vi "Start WiFi with DHCP.vi"(7 "Retry wait time [ms]":u32=100, 8 "Error In":errorcluster, 11 "LINX Resource":T2) -> (0 "error out":errorcluster, 2 "TCP Configuration Out":T1, 3 "LINX Resource Out":T2={"IO"=enum."Remote", "Interface"=enum."Serial", "LINX Device Config"={"Interface"=enum."Serial", "COM Port"="COM13", "TCP Configuration"={"IP Address"="", "Port"=0}, "Device Family"=1, "Device ID"=1, "Device Name"="myRIO-1900", "TCP Ref"=refnum, "Channels"={"DI"=[0, 1, 2, 3, 4, 5, 6, 7, 8, 9, 10, 11, 12, 13, 14, 15, 16, 17, 18, 19, 20, 21, 22, 23, 24, 25, 26, 27, 28, 29, 30, 31, 32, 33, 34, 35, 36, 37, 38, 39, 40, 41, 42, 43, 44, 45, 46], "DO"=[0, 1, 2, 3, 4, 5, 6, 7, 8, 9, 10, 11, 12, 13, 14, 15, 16, 17, 18, 19, 20, 21, 22, 23, 24, 25, 26, 27, 28, 29, 30, 31, 32, 33, 34, 35, 36, 37, 38, 39, 40, 41, 42, 43, 44, 45, 46], "AI"=[0, 1, 2, 3, 4, 5, 6, 7, 8, 9, 10, 11], "AO"=[], "PWM"=[3, 5, 6, 9, 10], "QE"=[], "UART"=[0, 1], "I2C 2"=[0], "SPI"=[0], "CAN"=[], "Servo"=[], "AI Ref (V)"=0.0, "AI Resolution (Bits)"=0, "AO Ref (V)"=0.0, "AO Resolution (Bits)"=0}}})   [LabVIEW 2019, in "LINXx.lvlib"]
doc: "Attempts to connect board to network with DHCP. Returns dynamically-assigned IP if successful"
uses:
  LINXx.lvlib
  <vilib>/MakerHub/LINX/Private/Type Defs/LINX Ref.ctl
  <vilib>/MakerHub/LINX/Private/Type Defs/Platform.ctl
  <vilib>/MakerHub/LINX/Private/Type Defs/Interface.ctl
  <vilib>/MakerHub/LINX/Private/Device/Type Defs/LINX Device Config.ctl
  <vilib>/MakerHub/LINX/Private/Device/Type Defs/TCP Config.ctl
  <vilib>/MakerHub/LINX/Private/Device/Type Defs/Channels.ctl
  <vilib>/MakerHub/LINX/Private/Device/Device.lvlib
  <vilib>/MakerHub/LINX/LMH-LINX.lvlib
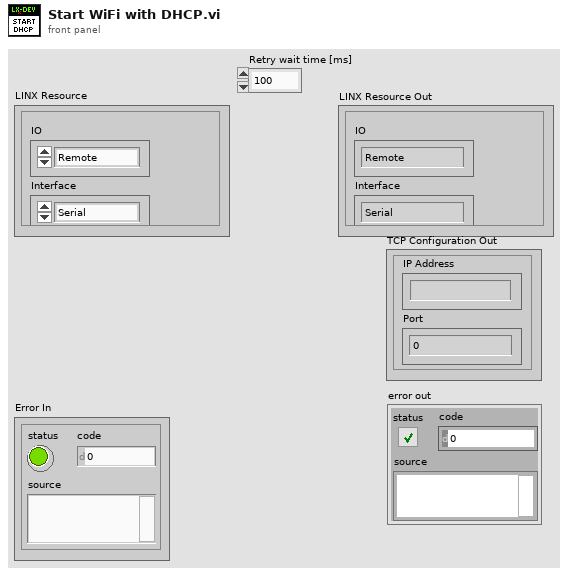
[diagram p1: front panel]
types:
  T1 = typedef "LMH-LINX.lvlib/Device.lvlib/TCP Config.ctl" = cluster{"IP Address":string, "Port":u16}
  T2 = typedef "LMH-LINX.lvlib/LINX Ref.ctl" = cluster{"IO":T3, "Interface":T4, "LINX Device Config":T5}
  T3 = typedef "LMH-LINX.lvlib/Platform.ctl" = enum16{"Remote", "Local"}
  T4 = typedef "LMH-LINX.lvlib/Interface.ctl" = enum16{"Serial", "TCP"}
  T5 = typedef "LMH-LINX.lvlib/Device.lvlib/LINX Device Config.ctl" = cluster{"Interface":T4, "COM Port":refnum<visa-resource-name>, "TCP Configuration":T1, "Device Family":u8, "Device ID":u8, "Device Name":string, "TCP Ref":refnum<k5>, "Channels":T6}
  T6 = typedef "LMH-LINX.lvlib/Channels.ctl" = cluster{"DI":u8[], "DO":u8[], "AI":u8[], "AO":u8[], "PWM":u8[], "QE":u8[], "UART":u8[], "I2C 2":u8[], "SPI":u8[], "CAN":u8[], "Servo":u8[], "AI Ref (V)":dbl, "AI Resolution (Bits)":u8, "AO Ref (V)":dbl, "AO Resolution (Bits)":u8}
  T7 = typedef "LMH-LINX.lvlib/Device.lvlib/Wifi Config.ctl" = cluster{"SSID":string, "IP Address":string, "Port":u16, "WIFI Security Type":T8, "Password":string}
  T8 = typedef "LMH-LINX.lvlib/WIFI Security Type.ctl" = enum8{"None", "WPA2 Password", "WPA2 Key", "WEP40", "WEP104"}
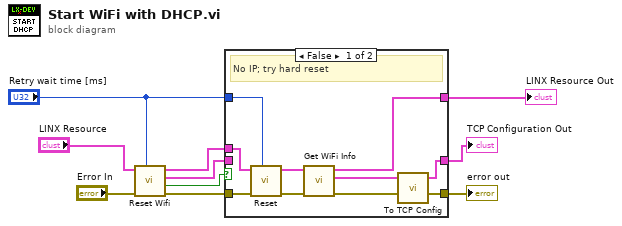
[diagram p0: block diagram]
diagram:
  n1 = call "Reset Wifi.vi"("Retry wait time [ms]"="Retry wait time [ms]", "error in (no error)"="Error In", "LINX Resource"="LINX Resource") -> ("error out"=w10:errorcluster, "Connected to network?"=w5:bool, "TCP Config"=w4:T1, "LINX Resource Out"=w7:T2)  [unwired: 5 in]
  n2 = case shown="False" w5 {
    tunnel: w10 -> [w19 w22]
    tunnel: [w13 w22] -> w1
    tunnel: w7 -> [w18 w21]
    tunnel: [w14 w21] -> w6
    tunnel: [w11 w20] -> w3
    tunnel: w4 -> [_ w20]
    tunnel: "Retry wait time [ms]" -> [w17 _]
    frame False {
      # "No IP; try hard reset"
      n3 = call "Reset.vi"("Reconnect \nwait time [ms]"=w17, "Error In"=w19, "LINX Resource"=w18) -> ("Error Out"=w16:errorcluster, "LINX Resource out"=w15:T2)  [unwired: 7 in]
      n4 = call "Get WiFi Info.vi"("Error In"=w16, "LINX Resource"=w15) -> ("Error Out"=w13:errorcluster, "WiFi Info"=w12:T7, "LINX Resource Out"=w14:T2)  [unwired: 6 in, 1 out]
      n5 = call "To TCP Config.vi"("Wifi Configuration"=w12) -> ("TCP Configuration"=w11:T1)  [unwired: 4 in]
    }
    frame True {
      # "Success, got new IP"
    }
  }
  "LINX Resource Out" <- w6
  "TCP Configuration Out" <- w3
  "error out" <- w1
